vi "gun_speed_mode_datastore.vi"(10 "data_store_mode":enum16{"Set", "Get"}(ring), 11 "Shooter Control Mode":T1) -> (3 "Shooter Control Mode Out":T1)   [LabVIEW 2011]
uses:
  gun_motor_state.ctl
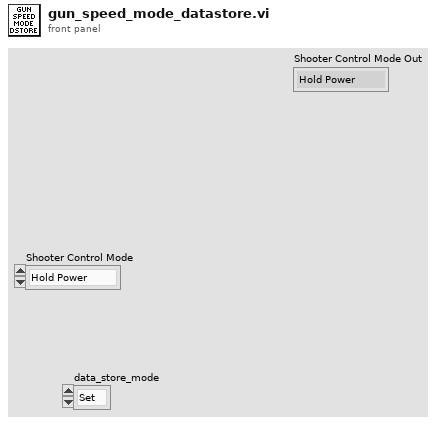
[diagram p1: front panel]
types:
  T1 = typedef "gun_motor_state.ctl" = enum16{"Hold Power", "Hold Speed", "Hold Distance", "Stop"}
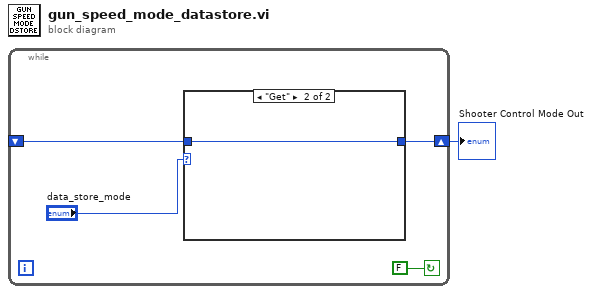
[diagram p0: block diagram]
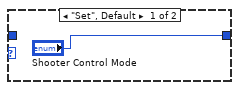
[diagram p2: hidden frame]
diagram:
  n1 = while {
    shift-right: [w3] -> w1
    shift-left: _ -> [w2]
    stop <- FALSE continue-if-true
    n2 = case shown="\"Get\"" "data_store_mode" {
      tunnel: ["Shooter Control Mode" w7] -> w3
      tunnel: w2 -> [_ w7]
      frame "Set", Default {
      }
      frame "Get" {
      }
    }
  }
  "Shooter Control Mode Out" <- w1
